vi "sub_ofdm_subcarrier_partitioner.vi"(8 "pilot carrier":i32, 9 "message carrier":i32, 10 "FFT size":i32, 11 "received symbol":cdb[](array[numeric])) -> (0 "pilot subcarriers":cdb[](array[numeric]), 3 "message subcarriers":cdb[](array[numeric]))   [LabVIEW 2014]
panel:
  out "size(s) 2":i32
  out "size(s)":i32
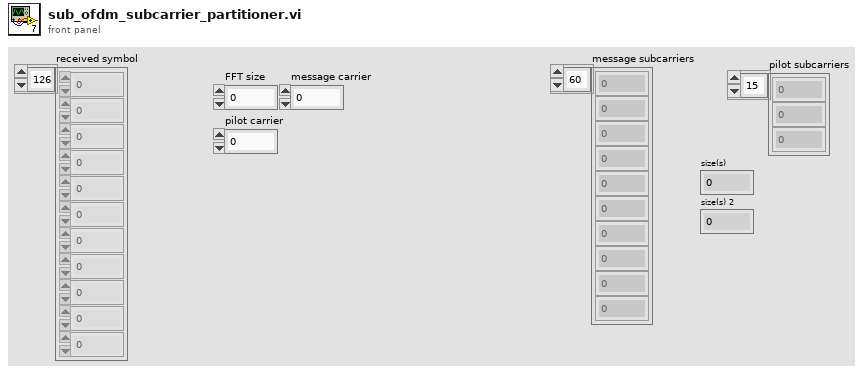
[diagram p1: front panel]
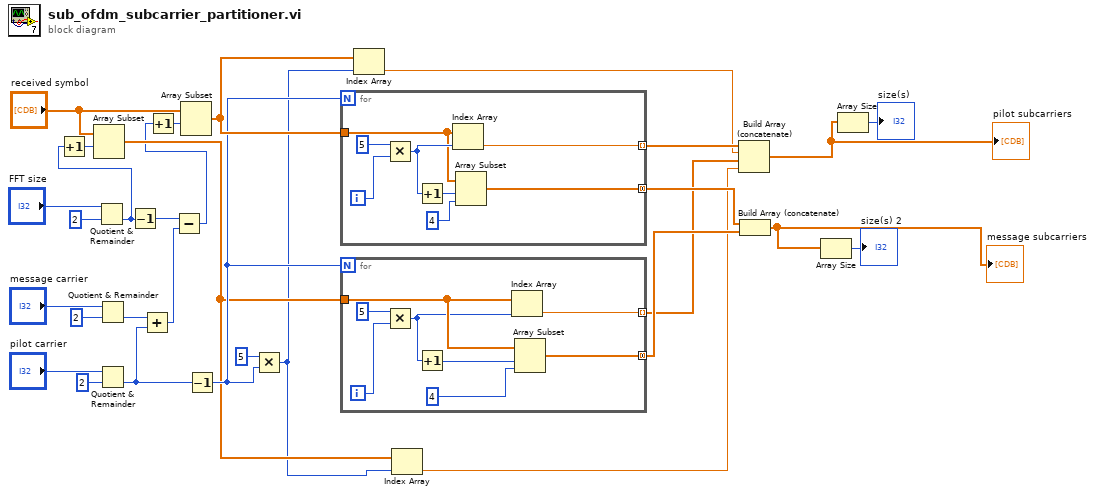
[diagram p0: block diagram]
diagram:
  n1 = Quotient & Remainder(x="FFT size", y=2) -> (floor(x/y)=w1:i32)  [unwired: 1 out]
  n2 = Increment(x=w1) -> (x+1=w2:i32)
  n3 = Array Subset(array="received symbol", index=w2) -> (w6:cdb[])  [unwired: 1 in]
  n4 = Quotient & Remainder(x="message carrier", y=2) -> (floor(x/y)=w17:i32)  [unwired: 1 out]
  n5 = Quotient & Remainder(x="pilot carrier", y=2) -> (floor(x/y)=w9:i32)  [unwired: 1 out]
  n6 = Decrement(x=w1) -> (x-1=w16:i32)
  n7 = Add(x=w17, y=w9) -> (x+y=w15:i32)
  n8 = Subtract(x=w16, y=w15) -> (x-y=w3:i32)
  n9 = Increment(x=w3) -> (x+1=w4:i32)
  n10 = Array Subset(array="received symbol", index=w4) -> (w14:cdb[])  [unwired: 1 in]
  n11 = Decrement(x=w9) -> (x-1=w8:i32)
  n12 = Multiply(x=5, y=w8) -> (x*y=w5:i32)
  n13 = for {
    N: w8 -> [_]
    tunnel: w14 -> [w34]
    tunnel: [w32] -> w26 mode=concatenating
    tunnel: [w31] -> w28 mode=indexing
    i -> [w37]
    n14 = Multiply(x=5, y=w37) -> (x*y=w35:i32)
    n15 = Increment(x=w35) -> (x+1=w36:i32)
    n16 = Index Array(array=w34, index=w35) -> (element=w31:cdb)
    n17 = Array Subset(array=w34, index=w36, length=4) -> (w32:cdb[])
  }
  n18 = for {
    N: w8 -> [_]
    tunnel: w6 -> [w44]
    tunnel: [w42] -> w24 mode=concatenating
    tunnel: [w41] -> w23 mode=indexing
    i -> [w45]
    n19 = Multiply(x=5, y=w45) -> (x*y=w40:i32)
    n20 = Increment(x=w40) -> (x+1=w39:i32)
    n21 = Index Array(array=w44, index=w40) -> (element=w41:cdb)
    n22 = Array Subset(array=w44, index=w39, length=4) -> (w42:cdb[])
  }
  n23 = Index Array(array=w14, index=w5) -> (element=w27:cdb)
  n24 = Index Array(array=w6, index=w5) -> (element=w22:cdb)
  n25 = Build Array (concatenate)(w28, w27, w23, w22) -> (w13:cdb[])
  "pilot subcarriers" <- w13
  n26 = Build Array (concatenate)(w26, w24) -> (w11:cdb[])
  "message subcarriers" <- w11
  n27 = Array Size(array=w11) -> (size(s)=→"size(s) 2":i32)
  n28 = Array Size(array=w13) -> (size(s)=→"size(s)":i32)
